vi "Calculate rectangle.vi"(8 "error in (no error)":errorcluster, 10 "xyzs array":dbl[](array[numeric]), 11 "Tomo in":refnum<class "Tomo.lvclass">) -> (0 "error out":errorcluster, 2 "rectangle":i32[](array[numeric]), 3 "Tomo out":refnum<class "Tomo.lvclass">)   [LabVIEW 2012, in "Tomo.lvclass"]
uses:
  Tomo.lvclass
  Tomo.lvclass/Tomo.ctl
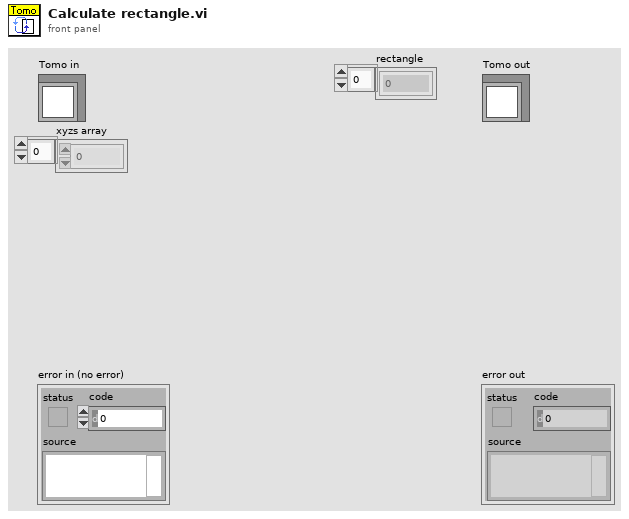
[diagram p1: front panel]
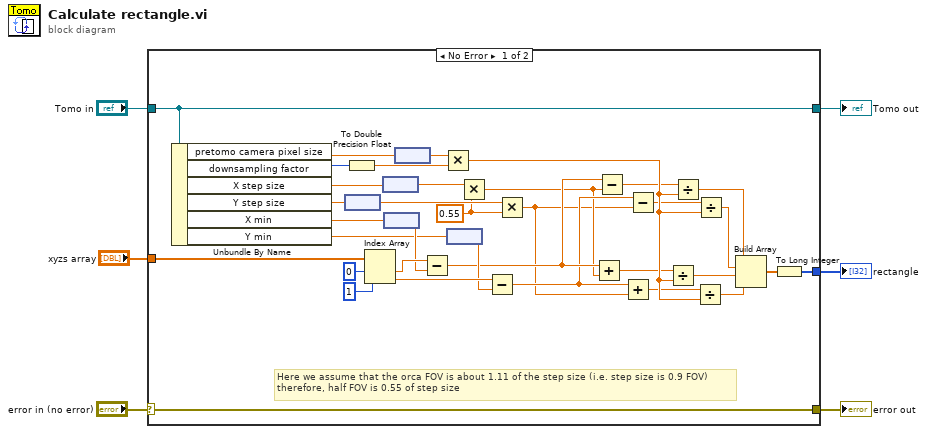
[diagram p0: block diagram]
diagram:
  n1 = case shown="No Error" "error in (no error)" {
    selector: "error in (no error)" -> [w41 w43]
    tunnel: [w41 w43] -> w5
    tunnel: [w40 w42] -> w3
    tunnel: "Tomo in" -> [w40 w42]
    tunnel: "xyzs array" -> [w39 _]
    tunnel: [w7 _] -> w1
    frame No Error {
      w23 = 0.55
      # "Here we assume that the orca FOV is about 1.11 of the step size (i.e. step size is 0.9 FOV)\ntherefore, half FOV is 0.55 of step size"
      n2 = Unbundle By Name(w40) -> ("pretomo camera pixel size"=w28:dbl[unit], "downsampling factor"=w30:u32, "X step size"=w27:dbl[unit], "Y step size"=w26:dbl[unit], "X min"=w35:dbl[unit], "Y min"=w33:dbl[unit])
      n3 = node(w26) -> (w24:dbl)
      n4 = To Double Precision Float(number=w30) -> (double precision float=w29:dbl)
      n5 = Index Array(array=w39, index #1=0 ("index"), index #2=1 ("index")) -> (element #1=w36:dbl, element #2=w32:dbl)
      n6 = node(w27) -> (w25:dbl)
      n7 = node(w35) -> (w34:dbl)
      n8 = node(w28) -> (w8:dbl)
      n9 = Subtract(x=w36, y=w34) -> (x-y=w22:dbl)
      n10 = Multiply(x=w8, y=w29) -> (x*y=w18:dbl)
      n11 = node(w33) -> (w31:dbl)
      n12 = Multiply(x=w25, y=w23) -> (x*y=w20:dbl)
      n13 = Subtract(x=w32, y=w31) -> (x-y=w21:dbl)
      n14 = Multiply(x=w24, y=w23) -> (x*y=w19:dbl)
      n15 = Add(x=w22, y=w20) -> (x+y=w15:dbl)
      n16 = Subtract(x=w22, y=w20) -> (x-y=w17:dbl)
      n17 = Add(x=w21, y=w19) -> (x+y=w14:dbl)
      n18 = Subtract(x=w21, y=w19) -> (x-y=w16:dbl)
      n19 = Divide(x=w15, y=w18) -> (x/y=w11:dbl)
      n20 = Divide(x=w17, y=w18) -> (x/y=w13:dbl)
      n21 = Divide(x=w14, y=w18) -> (x/y=w10:dbl)
      n22 = Divide(x=w16, y=w18) -> (x/y=w12:dbl)
      n23 = Build Array(w13, w12, w11, w10) -> (w9:dbl[])
      n24 = To Long Integer(number=w9) -> (32bit integer=w7:i32[])
    }
    frame Error {
    }
  }
  "error out" <- w5
  "Tomo out" <- w3
  "rectangle" <- w1
